vi "Configure Trigger (Delay).vi"(0 "VISA resource name":refnum<visa-resource-name>, 2 "Upper Limit (2E-6 s)":dbl=2e-06, 5 "Signal Source A (0: Channel 1)":i32(ring) items=["Channel 1", "Channel 2", "Channel 3", "Channel 4"], 7 "Signal Source B (0: Channel 1)":i32(ring)=1 items=["Channel 1", "Channel 2", "Channel 3", "Channel 4"], 9 "Edge Type (0: RTOR)":i32(ring) items=["RTOR", "RTOF", "FTOR", "FTOF"], 11 "error in (no error)":errorcluster, 12 "Delay Type (0: Greater)":i32(ring) items=["Greater", "Less", "InRange"], 13 "Lower Limit (1E-6 s)":dbl=1e-06, 14 "Trigger Level (0)":dbl) -> (4 "VISA resource name out":refnum<visa-resource-name>, 15 "error out":errorcluster)   [LabVIEW 2015, in "ZhiYuan ZDS Series for TCP.lvlib"]
doc: "Configures the setting for delay trigger.\n\nNote: This VI is only applicable for DS 2000 Series."
uses:
  ZhiYuan ZDS Series for TCP.lvlib
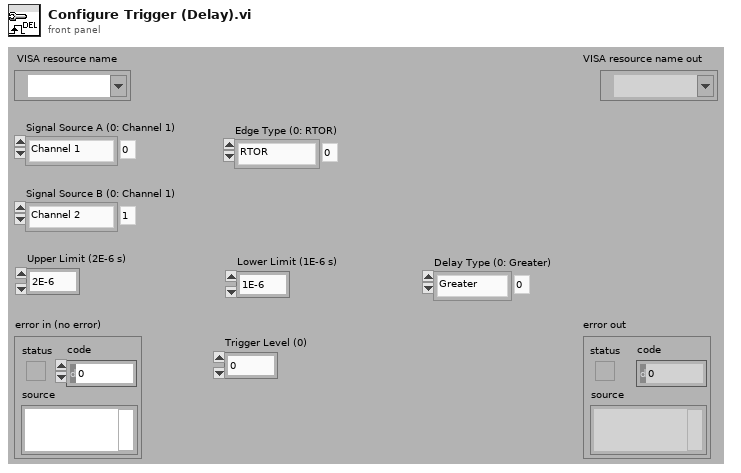
[diagram p1: front panel]
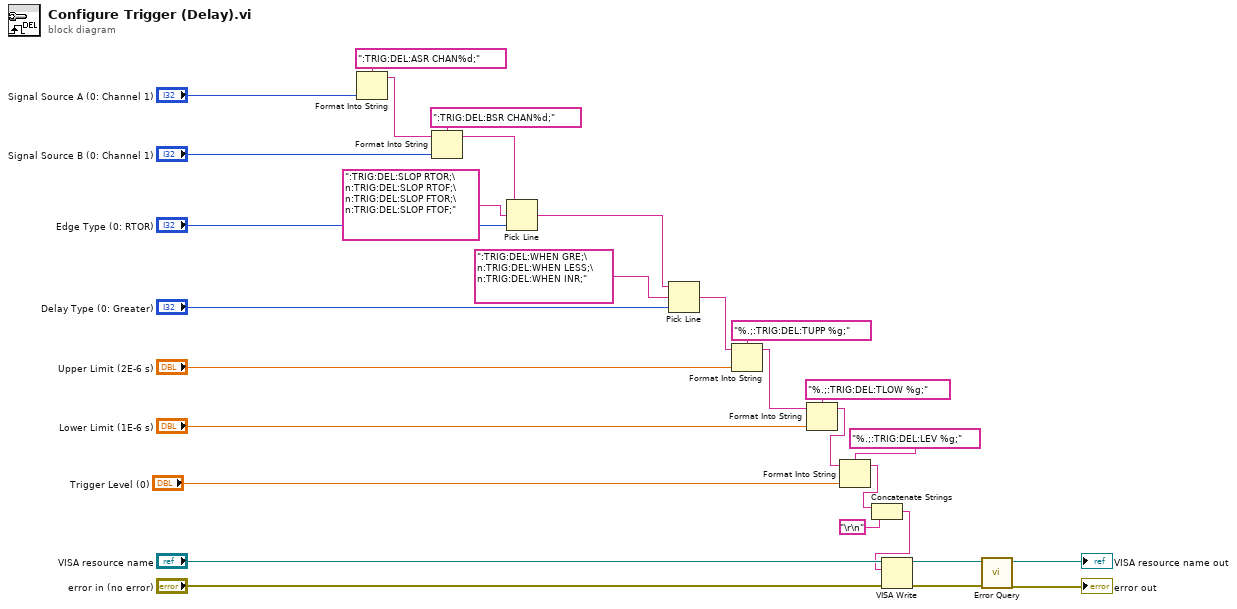
[diagram p0: block diagram]
diagram:
  n1 = Format Into String(format string=":TRIG:DEL:ASR CHAN%d;", "Signal Source A (0: Channel 1)") -> (resulting string=w27:string)  [unwired: 2 in, 1 out]
  n2 = Format Into String(format string=":TRIG:DEL:BSR CHAN%d;", initial string=w27, "Signal Source B (0: Channel 1)") -> (resulting string=w22:string)  [unwired: 1 in, 1 out]
  n3 = Pick Line(string ("")=w22, multi-line string=":TRIG:DEL:SLOP RTOR;\n:TRIG:DEL:SLOP RTOF;\n:TRIG:DEL:SLOP FTOR;\n:TRIG:DEL:SLOP FTOF;", line index="Edge Type (0: RTOR)") -> (output string=w7:string)
  n4 = Pick Line(string ("")=w7, multi-line string=":TRIG:DEL:WHEN GRE;\n:TRIG:DEL:WHEN LESS;\n:TRIG:DEL:WHEN INR;", line index="Delay Type (0: Greater)") -> (output string=w19:string)
  n5 = Format Into String(format string="%.;:TRIG:DEL:TUPP %g;", initial string=w19, "Upper Limit (2E-6 s)") -> (resulting string=w16:string)  [unwired: 1 in, 1 out]
  n6 = Format Into String(format string="%.;:TRIG:DEL:TLOW %g;", initial string=w16, "Lower Limit (1E-6 s)") -> (resulting string=w5:string)  [unwired: 1 in, 1 out]
  n7 = Format Into String(format string="%.;:TRIG:DEL:LEV %g;", initial string=w5, "Trigger Level (0)") -> (resulting string=w3:string)  [unwired: 1 in, 1 out]
  n8 = Concatenate Strings(w3, "\r\n") -> (w1:string)
  n9 = VISA Write(VISA resource name="VISA resource name", write buffer=w1, error in (no error)="error in (no error)") -> (VISA resource name out=w11:refnum<visa-resource-name>, error out=w10:errorcluster)  [unwired: 1 out]
  n10 = call "Error Query.vi"("error in (no error)"=w10, "VISA resource name"=w11) -> ("error out"=→"error out":errorcluster, "VISA resource name out"=→"VISA resource name out":refnum<visa-resource-name>)  [unwired: 6 in, 2 out]
